vi "Do.vi"(7 "Mediated Asynchronous Actor":refnum<class "Mediated Asynchronous Actor.lvclass">, 8 "error in (no error)":errorcluster, 11 "Write Msg in":refnum<class "Write Msg.lvclass">) -> (0 "error out":errorcluster, 3 "Write Msg out":refnum<class "Write Msg.lvclass">, 5 "Mediated Asynchronous Actor out":refnum<class "Mediated Asynchronous Actor.lvclass">)   [LabVIEW 2016, in "Stream Mediator.lvlib" / "Write Msg.lvclass"]
doc: "--\nCopyright © 2017 Composed SystemsI All rights reserved.\n\nAuthor: Jon McBee <jon.mcbee@composed.io>\n\nThis library is provided \"AS IS\" ,WITHOUT WARRANTIES OR\nCONDITIONS OF ANY KIND, either express or implied.\n\nComposed Systems -- composed.io\n\nStream 0.0.1.1\nJon McBee - Composed Systems\nCopyright (c) 2017, Composed Systems"
uses:
  <userlib>/Composed Systems/Stream/Mediator/Classes/Websocket Client Handler Actor/Websocket Client Handler Msgs/Write Msg/Write Msg.lvclass
  <userlib>/Composed Systems/Stream/Mediator/Classes/Mediated Asynchronous Actor/Mediated Asynchronous Actor.lvclass
  <userlib>/Composed Systems/Stream/Mediator/Classes/Websocket Client Handler Actor/Websocket Client Handler/Websocket Client Handler.lvclass
  C:/Program Files (x86)/National Instruments/LabVIEW 2016/user.lib/Composed Systems/Stream/Mediator/Classes/Mediated Asynchronous Actor/Mediated Asynchronous Actor.lvclass
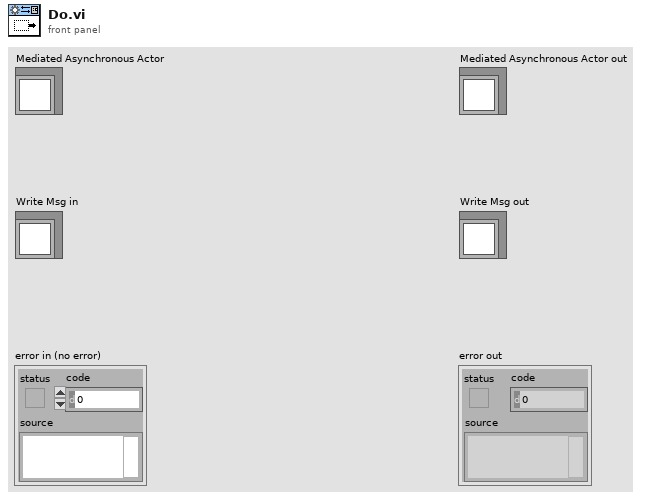
[diagram p1: front panel]
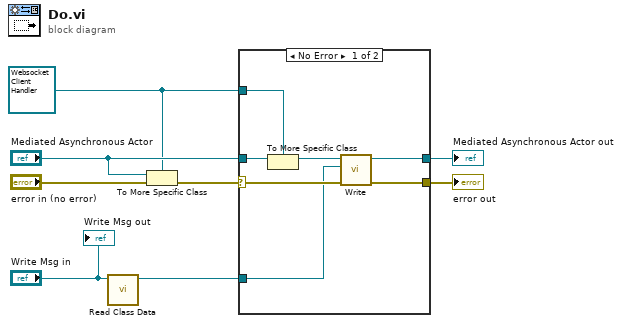
[diagram p0: block diagram]
diagram:
  w5 = refnum<class "Websocket Client Handler.lvclass"> refnum ("Websocket Client Handler.lvclass")
  n1 = call <userlib>:"Read Class Data.vi"("Write Msg in"="Write Msg in") -> ("Message"=w1:refnum<class "Message Interface.lvclass">)  [unwired: 9 in, 1 out]
  n2 = To More Specific Class(target class=w5, reference="Mediated Asynchronous Actor", error in="error in (no error)") -> (error out=w7:errorcluster)  [unwired: 1 out]
  n3 = case shown="No Error" w7 {
    selector: w7 -> [w15 w16]
    tunnel: "Mediated Asynchronous Actor" -> [w13 w17]
    tunnel: w5 -> [w12 _]
    tunnel: [w11 w16] -> w4
    tunnel: [w10 w17] -> w3
    tunnel: w1 -> [w9 _]
    frame No Error {
      n4 = To More Specific Class(target class=w12, reference=w13) -> (specific class reference=w14:refnum<class "Websocket Client Handler.lvclass">)  [unwired: 1 in, 1 out]
      n5 = call <userlib>:"Write.vi"("error in (no error)"=w15, "Message"=w9, "Websocket Client Handler in"=w14) -> ("error out"=w11:errorcluster, "Websocket Client Handler out"=w10:refnum<class "Websocket Client Handler.lvclass">)  [unwired: 7 in]
    }
    frame Error {
    }
  }
  "error out" <- w4
  "Mediated Asynchronous Actor out" <- w3
  "Write Msg out" <- "Write Msg in"
